vi "OP600ZP_FDT_V2.vi"(8 "errin":errorcluster) -> (0 "errout":errorcluster, 2 "Log":string, 3 "is OK?":bool)   [LabVIEW 2020]
uses:
  VG/Ubatt.vi
  VG/PackType.vi
  VG/IS30%.vi
  OP600ZP_VGConf.vi
panel:
  out "PASS/FAIL?":string
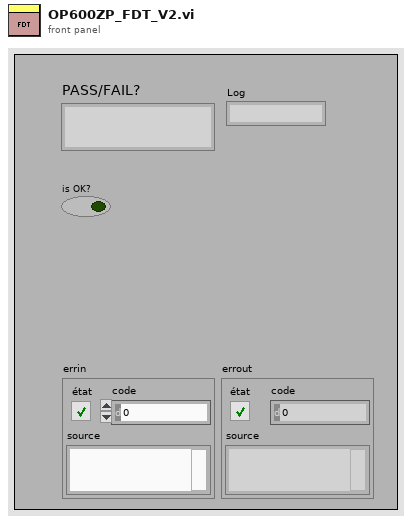
[diagram p1: front panel]
types:
  T1 = cluster{string, string, string, string, string, string, string, string, string, string}
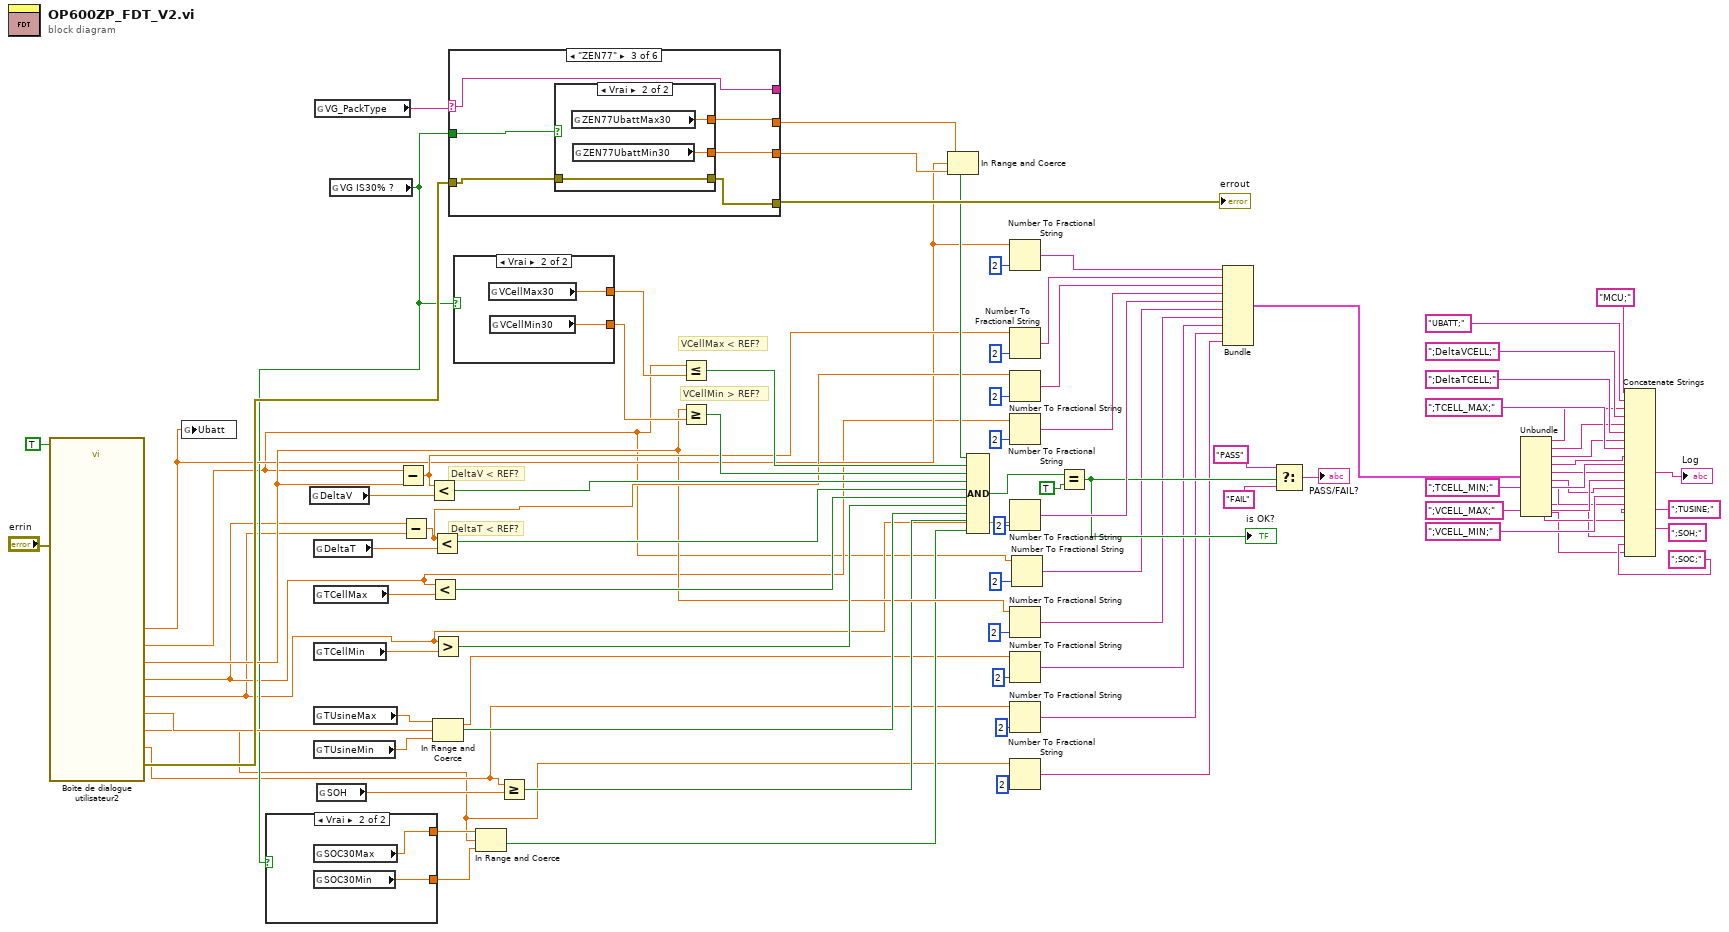
[diagram p0: block diagram]
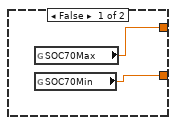
[diagram p2: hidden frame]
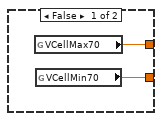
[diagram p3: hidden frame]
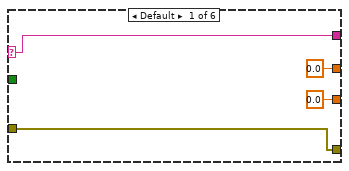
[diagram p4: hidden frame]
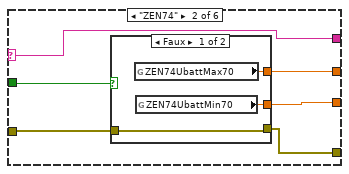
[diagram p5: hidden frame]
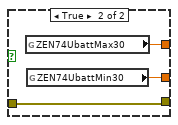
[diagram p6: hidden frame]
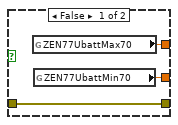
[diagram p7: hidden frame]
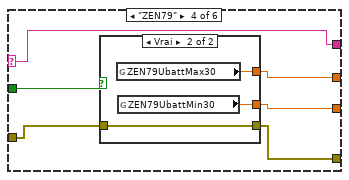
[diagram p8: hidden frame]
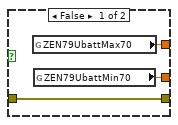
[diagram p9: hidden frame]
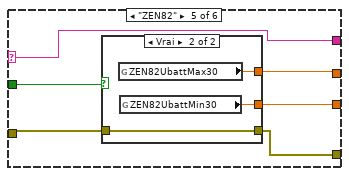
[diagram p10: hidden frame]
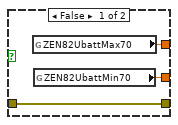
[diagram p11: hidden frame]
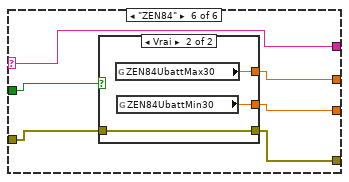
[diagram p12: hidden frame]
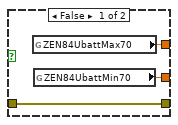
[diagram p13: hidden frame]
diagram:
  # "DeltaT < REF?"
  # "DeltaV < REF?"
  # "VCellMin > REF?"
  # "VCellMax < REF?"
  n1 = call "Boîte de dialogue utilisateur2"("Enable"=TRUE, "error in (no error)"="errin") -> ("SOH"=w16:dbl, "SOC"=w14:dbl, "Factory Temperature"=w27:dbl, "Min Cell Temperature"=w5:dbl, "Max Cell Temperature"=w7:dbl, "Min Cell Voltage"=w26:dbl, "Max Cell Voltage"=w2:dbl, "Battery Voltage"=w25:dbl, "error out"=w28:errorcluster)  [unwired: 7 in, 2 out]
  n2 = global write "Ubatt.vi" "Ubatt"(w25) -> ()
  n3 = global read "OP600ZP_VGConf.vi" "DeltaV"() -> (w74:dbl)
  n4 = global read "OP600ZP_VGConf.vi" "DeltaT"() -> (w73:dbl)
  n5 = global read "OP600ZP_VGConf.vi" "TCellMax"() -> (w66:dbl)
  n6 = global read "OP600ZP_VGConf.vi" "TCellMin"() -> (w67:dbl)
  n7 = global read "OP600ZP_VGConf.vi" "TUsineMax"() -> (w59:dbl)
  n8 = global read "OP600ZP_VGConf.vi" "TUsineMin"() -> (w58:dbl)
  n9 = global read "PackType.vi" "VG_PackType"() -> (w89:string)
  n10 = global read "OP600ZP_VGConf.vi" "SOH"() -> (w19:dbl)
  n11 = global read "IS30%.vi" "VG IS30% ?"() -> (w22:bool)
  n12 = case shown="Vrai" w22 {
    tunnel: [w91 w93] -> w21
    tunnel: [w90 w92] -> w20
    frame False {
      n13 = global read "OP600ZP_VGConf.vi" "SOC70Max"() -> (w91:dbl)
      n14 = global read "OP600ZP_VGConf.vi" "SOC70Min"() -> (w90:dbl)
    }
    frame True {
      n15 = global read "OP600ZP_VGConf.vi" "SOC30Max"() -> (w93:dbl)
      n16 = global read "OP600ZP_VGConf.vi" "SOC30Min"() -> (w92:dbl)
    }
  }
  n17 = Subtract(x=w2, y=w26) -> (x-y=w63:dbl)
  n18 = Subtract(x=w7, y=w5) -> (x-y=w62:dbl)
  n19 = Less?(x=w63, y=w74) -> (x < y?=w71:bool)
  n20 = Less?(x=w7, y=w66) -> (x < y?=w65:bool)
  n21 = Less?(x=w62, y=w73) -> (x < y?=w72:bool)
  n22 = Greater?(x=w5, y=w67) -> (0:w64:bool)
  n23 = In Range and Coerce(upper limit=w59, x=w27, lower limit=w58) -> (coerced(x)=w6:dbl, In Range?=w57:bool)
  n24 = case shown="\"ZEN77\"" w89 {
    selector: w89 -> [w97 w100 w112 w124 w136 w148]
    tunnel: [0.0 ("ZEN84UbattMax30") w103 w115 w127 w139 w151] -> w75
    tunnel: [0.0 ("ZEN84UbattMin30") w102 w114 w126 w138 w150] -> w76
    tunnel: w22 -> [_ w101 w113 w125 w137 w149]
    tunnel: [w97 w100 w112 w124 w136 w148] -> _
    tunnel: w28 -> [w96 w99 w111 w123 w135 w147]
    tunnel: [w96 w98 w110 w122 w134 w146] -> w88
    frame Default {
    }
    frame "ZEN74" {
      n25 = case shown="Faux" w101 {
        tunnel: [w106 w109] -> w103
        tunnel: [w105 w108] -> w102
        tunnel: [w104 w107] -> w98
        tunnel: w99 -> [w104 w107]
        frame False {
          n26 = global read "OP600ZP_VGConf.vi" "ZEN74UbattMax70"() -> (w106:dbl)
          n27 = global read "OP600ZP_VGConf.vi" "ZEN74UbattMin70"() -> (w105:dbl)
        }
        frame True {
          n28 = global read "OP600ZP_VGConf.vi" "ZEN74UbattMax30"() -> (w109:dbl)
          n29 = global read "OP600ZP_VGConf.vi" "ZEN74UbattMin30"() -> (w108:dbl)
        }
      }
    }
    frame "ZEN77" {
      n30 = case shown="Vrai" w113 {
        tunnel: [w118 w121] -> w115
        tunnel: [w117 w120] -> w114
        tunnel: w111 -> [w116 w119]
        tunnel: [w116 w119] -> w110
        frame False {
          n31 = global read "OP600ZP_VGConf.vi" "ZEN77UbattMax70"() -> (w118:dbl)
          n32 = global read "OP600ZP_VGConf.vi" "ZEN77UbattMin70"() -> (w117:dbl)
        }
        frame True {
          n33 = global read "OP600ZP_VGConf.vi" "ZEN77UbattMax30"() -> (w121:dbl)
          n34 = global read "OP600ZP_VGConf.vi" "ZEN77UbattMin30"() -> (w120:dbl)
        }
      }
    }
    frame "ZEN79" {
      n35 = case shown="Vrai" w125 {
        tunnel: [w130 w133] -> w127
        tunnel: [w129 w132] -> w126
        tunnel: w123 -> [w128 w131]
        tunnel: [w128 w131] -> w122
        frame False {
          n36 = global read "OP600ZP_VGConf.vi" "ZEN79UbattMax70"() -> (w130:dbl)
          n37 = global read "OP600ZP_VGConf.vi" "ZEN79UbattMin70"() -> (w129:dbl)
        }
        frame True {
          n38 = global read "OP600ZP_VGConf.vi" "ZEN79UbattMax30"() -> (w133:dbl)
          n39 = global read "OP600ZP_VGConf.vi" "ZEN79UbattMin30"() -> (w132:dbl)
        }
      }
    }
    frame "ZEN82" {
      n40 = case shown="Vrai" w137 {
        tunnel: [w142 w145] -> w139
        tunnel: [w141 w144] -> w138
        tunnel: w135 -> [w140 w143]
        tunnel: [w140 w143] -> w134
        frame False {
          n41 = global read "OP600ZP_VGConf.vi" "ZEN82UbattMax70"() -> (w142:dbl)
          n42 = global read "OP600ZP_VGConf.vi" "ZEN82UbattMin70"() -> (w141:dbl)
        }
        frame True {
          n43 = global read "OP600ZP_VGConf.vi" "ZEN82UbattMax30"() -> (w145:dbl)
          n44 = global read "OP600ZP_VGConf.vi" "ZEN82UbattMin30"() -> (w144:dbl)
        }
      }
    }
    frame "ZEN84" {
      n45 = case shown="Vrai" w149 {
        tunnel: [w154 w157] -> w151
        tunnel: [w153 w156] -> w150
        tunnel: w147 -> [w152 w155]
        tunnel: [w152 w155] -> w146
        frame False {
          n46 = global read "OP600ZP_VGConf.vi" "ZEN84UbattMax70"() -> (w154:dbl)
          n47 = global read "OP600ZP_VGConf.vi" "ZEN84UbattMin70"() -> (w153:dbl)
        }
        frame True {
          n48 = global read "OP600ZP_VGConf.vi" "ZEN84UbattMax30"() -> (w157:dbl)
          n49 = global read "OP600ZP_VGConf.vi" "ZEN84UbattMin30"() -> (w156:dbl)
        }
      }
    }
  }
  "errout" <- w88
  n50 = case shown="Vrai" w22 {
    tunnel: [w159 w161] -> w4
    tunnel: [w158 w160] -> w61
    frame False {
      n51 = global read "OP600ZP_VGConf.vi" "VCellMax70"() -> (w159:dbl)
      n52 = global read "OP600ZP_VGConf.vi" "VCellMin70"() -> (w158:dbl)
    }
    frame True {
      n53 = global read "OP600ZP_VGConf.vi" "VCellMax30"() -> (w161:dbl)
      n54 = global read "OP600ZP_VGConf.vi" "VCellMin30"() -> (w160:dbl)
    }
  }
  n55 = In Range and Coerce(upper limit=w21, x=w14, lower limit=w20) -> (In Range?=w17:bool)  [unwired: 1 out]
  n56 = Greater Or Equal?(x=w16, y=w19) -> (x >= y?=w18:bool)
  n57 = Less Or Equal?(x=w2, y=w4) -> (x <= y?=w69:bool)
  n58 = Greater Or Equal?(x=w26, y=w61) -> (x >= y?=w70:bool)
  n59 = In Range and Coerce(upper limit=w75, x=w25, lower limit=w76) -> (In Range?=w68:bool)  [unwired: 1 out]
  n60 = Compound Arithmetic op=AND ("Opérateur arithmétique")(w68, w69, w70, w71, w72, w65, w64, w57, w18, w17) -> (w82:bool)
  n61 = Number To Fractional String(number=w25, precision (6)=i16 2 ("précision (6)")) -> (F-format string=w87:string)  [unwired: 2 in]
  n62 = Number To Fractional String(number=w63, precision (6)=i16 2 ("précision (6)")) -> (F-format string=w86:string)  [unwired: 2 in]
  n63 = Number To Fractional String(number=w62, precision (6)=i16 2 ("précision (6)")) -> (F-format string=w85:string)  [unwired: 2 in]
  n64 = Number To Fractional String(number=w7, precision (6)=i16 2 ("précision (6)")) -> (F-format string=w84:string)  [unwired: 2 in]
  n65 = Number To Fractional String(number=w5, precision (6)=i16 2 ("précision (6)")) -> (F-format string=w83:string)  [unwired: 2 in]
  n66 = Number To Fractional String(number=w26, precision (6)=i16 2 ("précision (6)")) -> (F-format string=w60:string)  [unwired: 2 in]
  n67 = Number To Fractional String(number=w6, precision (6)=i16 2 ("précision (6)")) -> (F-format string=w56:string)  [unwired: 2 in]
  n68 = Number To Fractional String(number=w16, precision (6)=i16 2 ("précision (6)")) -> (F-format string=w15:string)  [unwired: 2 in]
  n69 = Number To Fractional String(number=w14, precision (6)=i16 2 ("précision (6)")) -> (F-format string=w13:string)  [unwired: 2 in]
  n70 = Number To Fractional String(number=w2, precision (6)=i16 2 ("précision (6)")) -> (F-format string=w3:string)  [unwired: 2 in]
  n71 = Equal?(x=w82, y=TRUE) -> (x = y?=w78:bool)
  "is OK?" <- w78
  n72 = Bundle(w87, w86, w85, w84, w83, w3, w60, w56, w15, w13) -> (w31:T1)  [unwired: 1 in]
  n73 = Select ("Sélectionner")(t="PASS", s=w78, f="FAIL") -> (s? t:f=→"PASS/FAIL?":string)
  n74 = Unbundle(w31) -> (w40:string, w39:string, w38:string, w37:string, w36:string, w35:string, w34:string, w32:string, w11:string, w9:string)
  n75 = Concatenate Strings("MCU;" ("chaîne"), "UBATT;", w40, ";DeltaVCELL;", w39, ";DeltaTCELL;", w38, ";TCELL_MAX;", w37, ";TCELL_MIN;", w36, ";VCELL_MAX;", w35, ";VCELL_MIN;", w34, ";TUSINE;" ("chaîne"), w32, ";SOH;" ("chaîne"), w11, ";SOC;" ("chaîne"), w9) -> (→"Log":string)
